vi "Copy-template-image-folder.vi"(8 "error in":errorcluster, 11 "target path (use dialog)":path) -> (0 "error out":errorcluster)   [LabVIEW 2014]
panel:
  out "new path":path
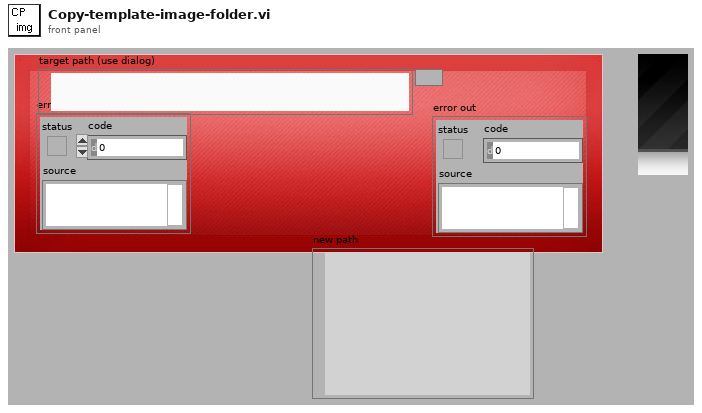
[diagram p1: front panel]
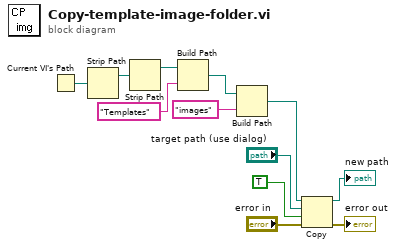
[diagram p0: block diagram]
diagram:
  n1 = Current VI's Path() -> (path=w12:path)
  n2 = Strip Path(path=w12) -> (stripped path=w11:path)  [unwired: 1 out]
  n3 = Strip Path(path=w11) -> (stripped path=w10:path)  [unwired: 1 out]
  n4 = Build Path(base path=w10, name or relative path="Templates") -> (appended path=w8:path)
  n5 = Build Path(base path=w8, name or relative path="images") -> (appended path=w7:path)
  n6 = Copy(8:"error in", 9:TRUE ("overwrite (F)"), 10:"target path (use dialog)", 11:w7) -> (0:→"error out":errorcluster, 3:→"new path":path)  [unwired: 2 out]
